vi "get_spectrum.vi"(11 "File (SHG Spectra)":path) -> (2 "Spectrum":dbl[](array[numeric]), 3 "Path":path)   [LabVIEW 2019]
uses:
  <vilib>/Utility/file.llb/Read Delimited Spreadsheet (DBL).vi
panel:
  out "all rows":dbl[][](array[numeric])
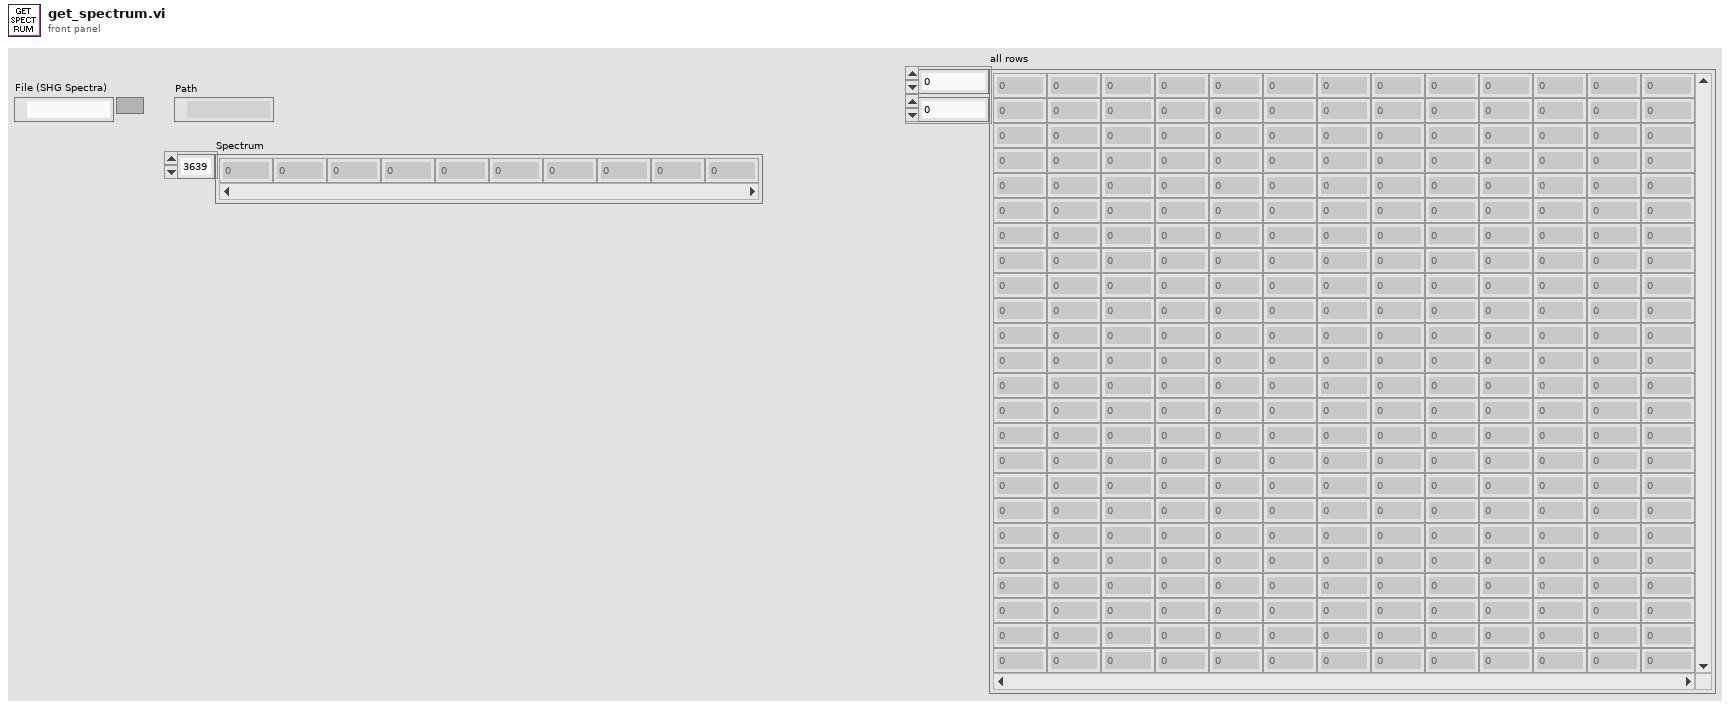
[diagram p1: front panel]
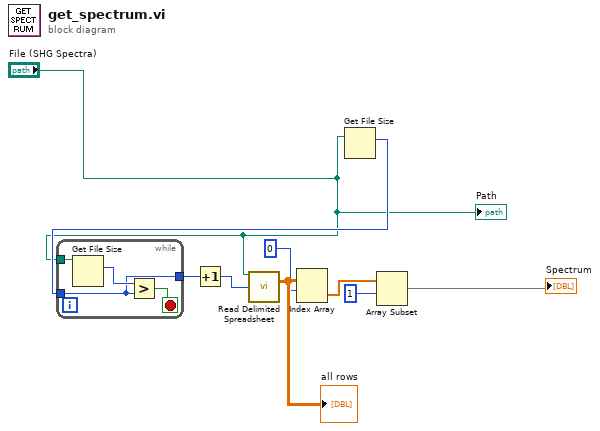
[diagram p0: block diagram]
diagram:
  n1 = Get File Size(file="File (SHG Spectra)") -> (size (in bytes)=w2:i64)  [unwired: 1 in, 2 out]
  n2 = while {
    tunnel: w2 -> [w11]
    tunnel: [w11] -> w3
    tunnel: "File (SHG Spectra)" -> [w10]
    stop <- w12 stop-if-true
    n3 = Get File Size(file=w10) -> (size (in bytes)=w13:i64)  [unwired: 1 in, 2 out]
    n4 = Greater?(x=w13, y=w11) -> (0:w12:bool)
  }
  n5 = Increment(x=w3) -> (x+1=w4:i64)
  n6 = call-poly <vilib>:"Read Delimited Spreadsheet.vi"("file path (dialog if empty)"="File (SHG Spectra)", "start of read offset (chars.:0)"=w4) -> ("all rows"=w7:dbl[][])  [unwired: 8 in, 5 out]
  "all rows" <- w7
  n7 = Index Array(array=w7, index (row)=0) -> (element=w8:dbl[])  [unwired: 1 in]
  n8 = Array Subset(array=w8, index=1) -> (→"Spectrum":dbl[])  [unwired: 1 in]
  "Path" <- "File (SHG Spectra)"
